vi "Begin.vi"(8 "error in":errorcluster) -> (0 "error out":errorcluster)   [LabVIEW 2015]
doc: "Called before other user functions, this VI is expected to open initial I/O refnums, load in file data, and do all program initialization. Notice that the <B>error out</B> terminal is simply used for data flow. Wiring it to other structures or subVIs ensures that this VI runs first."
uses:
  <vilib>/Rock Robotics/WPI/DriverStation/WPI_DriverStationRobotMode2.ctl
  <vilib>/Rock Robotics/WPI/Joystick/WPI_JoystickDeviceEnum.ctl
  <vilib>/Rock Robotics/SystemInterfaces/DIO/FPGA_DIOPWMChannel.ctl
  <vilib>/Rock Robotics/SystemInterfaces/DIO/FPGA_DIOChannel.ctl
  <vilib>/Rock Robotics/SystemInterfaces/DIO/FPGA_DIORelayChannel.ctl
  <vilib>/Rock Robotics/WPI/Camera/WPI_CameraExposure Values.ctl
  <vilib>/Rock Robotics/WPI/Camera/WPI_CameraWhite Balance Values.ctl
  <vilib>/Rock Robotics/WPI/Camera/WPI_CameraFrameRate.ctl
  <vilib>/Rock Robotics/WPI/Camera/WPI_CameraImageSize.ctl
  Robot Global Data.vi
  <vilib>/Rock Robotics/Network Tables/NT Write String Array.vi
  <vilib>/Rock Robotics/WPI/MotorControl/WPI_MotorControlOpen Talon.vi
  <vilib>/Rock Robotics/WPI/MotorControl/WPI_MotorControlOpen Victor.vi
  <vilib>/Rock Robotics/Network Tables/NT Write String.vi
  SubSystems/References/Refnums.vi
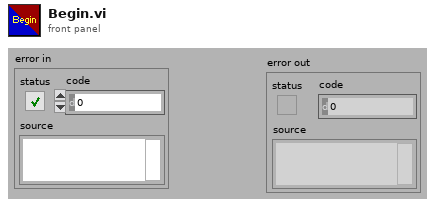
[diagram p1: front panel]
types:
  T1 = typedef "WPI_CameraImageSize.ctl" = enum16{"640x480", "320x240", "160x120", "Custom"}
  T2 = typedef "WPI_CameraFrameRate.ctl" = u32
  T3 = typedef "WPI_CameraExposure Values.ctl" = enum16{"Auto", "Flicker-free 50 Hz", "Flicker-free 60 Hz", "Hold current", "Custom"}
  T4 = typedef "WPI_CameraWhite Balance Values.ctl" = enum16{"Auto", "Fixed indoor", "Fixed outdoor 1", "Fixed outdoor 2", "Fixed fluorescent 1", "Fixed fluorescent 2", "Hold current", "Custom"}
  T5 = typedef "FPGA_DIORelayChannel.ctl" = enum8{"Relay 0", "Relay 1", "Relay 2", "Relay 3", "Invalid"}
  T6 = typedef "FPGA_DIOChannel.ctl" = enum8{"DIO 0", "DIO 1", "DIO 2", "DIO 3", "DIO 4", "DIO 5", "DIO 6", "DIO 7", "DIO 8", "DIO 9", "DIO MXP 0", "DIO MXP 1", "DIO MXP 2", "DIO MXP 3", "DIO MXP 4", "DIO MXP 5", "DIO MXP 6", "DIO MXP 7", "DIO MXP 8", "DIO MXP 9", "DIO MXP 10", "DIO MXP 11", "DIO MXP 12", "DIO MXP 13", "DIO MXP 14", "DIO MXP 15", "Invalid"}
  T7 = typedef "WPI_JoystickDeviceEnum.ctl" = enum16{"USB 0", "USB 1", "USB 2", "USB 3", "USB 4", "USB 5"}
  T8 = typedef "FPGA_DIOPWMChannel.ctl" = enum8{"PWM 0", "PWM 1", "PWM 2", "PWM 3", "PWM 4", "PWM 5", "PWM 6", "PWM 7", "PWM 8", "PWM 9", "PWM MXP 0", "PWM MXP 1", "PWM MXP 2", "PWM MXP 3", "PWM MXP 4", "PWM MXP 5", "PWM MXP 6", "PWM MXP 7", "PWM MXP 8", "PWM MXP 9", "Invalid"}
  T9 = typedef "WPI_DriverStationRobotMode2.ctl" = enum16{"Autonomous Disabled", "Autonomous Enabled", "Teleop Disabled", "Teleop Enabled", "Disconnected", "Finish", "Test Disabled", "Test Enabled", "Emergency Stopped"}
  T10 = typedef "WPI_JoystickDevRef.ctl" = cluster{"Device":T7}
  T11 = typedef "WPI_MotorControlDeviceRef.ctl" = cluster{"DeviceStatus":errorcluster, "Type":T12, "PWM":cluster{"PWM Channel":T8, "DeadBand":T13}, "CAN":cluster{"Device Number":u8, "Control Mode":T14, "Semaphore":T15, "Max Vout":dbl, "TalonSRX Control Mode":T16}, "Invert":bool}
  T12 = typedef "WPI_MotorControlType.ctl" = enum16{"PWM", "CAN", "CANTalonSRX"}
  T13 = typedef "WPI_PWMDeadband.ctl" = cluster{"Name":string, "maxPositivePwm":i32, "minPositivePwm":i32, "centerPwm":i32, "maxNegativePwm":i32, "minNegativePwm":i32, "angularRange":u16}
  T14 = typedef "WPI_CANJaguar_ControlMode.ctl" = enum8{"Percent VBus", "Current", "Speed", "Position", "Voltage"}
  T15 = typedef "Semaphore RefNum" = refnum<k1>
  T16 = typedef "WPI_CANTalonSRX_APIControlMode.ctl" = enum8{"Percent VBus", "Speed", "Position", "Slave", "Unchanged / Invalid", "Voltage Compensation", "Current", "Motion Profile"}
  T17 = typedef "WPI_RelayDevRef.ctl" = cluster{"DevStatus":errorcluster, "Relay Channel":T5, "Relay Direction":T18}
  T18 = typedef "WPI_RelayDirection.ctl" = enum16{"Both directions", "Forward only", "Reverse only"}
  T19 = typedef "WPI_CameraDevRef.ctl" = cluster{"Camera Address":string, "CameraStatus":errorcluster}
  T20 = typedef "WPI_DigitalInputDevRef.ctl" = cluster{"DevStatus":errorcluster, "DIO Channel":T6}
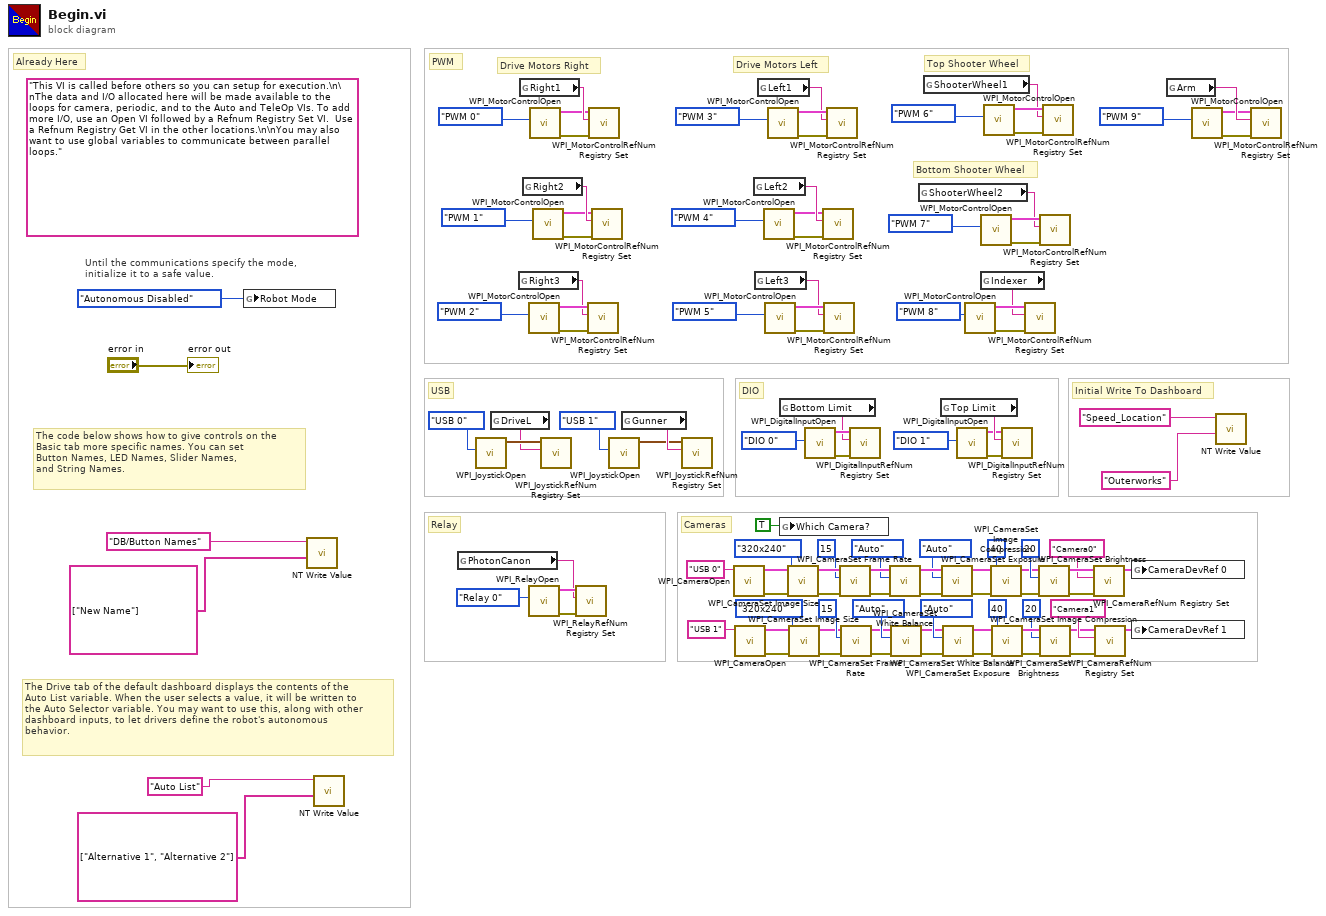
[diagram p0: block diagram]
diagram:
  (unwired) "This VI is called before others so you can setup for execution.\n\nThe data and I/O allocated here will be made available to the loops for camera, periodic, and to the Auto and TeleOp VIs. To add more I/O, use an Open VI followed by a Refnum Registry Set VI.  Use a Refnum Registry Get VI in the other locations.\n\nYou may also want to use global variables to communicate between parallel loops."
  # "Cameras"
  # "Initial Write To Dashboard"
  # "Bottom Shooter Wheel"
  # "Top Shooter Wheel"
  # "Drive Motors Left"
  # "Drive Motors Right"
  # "Relay"
  # "DIO"
  # "PWM"
  # "Already Here"
  # "USB"
  # "The Drive tab of the default dashboard displays the contents of the\nAuto List variable. When the user selects a value, it will be written to\nthe Auto Selector variable. You may want to use this, along with other\ndashboard inputs, to let drivers define the robot's autonomous\nbehavior."
  # "The code below shows how to give controls on the\nBasic tab more specific names. You can set\nButton Names, LED Names, Slider Names,\nand String Names."
  # "Until the communications specify the mode,\ninitialize it to a safe value."
  n1 = global write "Robot Global Data.vi" "Robot Mode"(WPI_DriverStationRobotMode2."Autonomous Disabled" ("Robot Mode")) -> ()
  n2 = call-poly <vilib>:"NT Write Value.vi"("String Array"=string[] ["New Name"], "Name"="DB/Button Names") -> ()  [unwired: 9 in, 1 out]
  n3 = call-poly <vilib>:"NT Write Value.vi"("String Array"=string[] ["Alternative 1", "Alternative 2"], "Name"="Auto List") -> ()  [unwired: 9 in, 1 out]
  n4 = global read "Refnums.vi" "PhotonCanon"() -> (w50:string)
  n5 = call <vilib>:"WPI_JoystickOpen.vi"("JoystickDevice"=WPI_JoystickDeviceEnum."USB 0") -> ("JoystickDevRef"=w107:T10)  [unwired: 10 in]
  n6 = global read "Refnums.vi" "DriveL"() -> (w106:string)
  n7 = global read "Refnums.vi" "Right3"() -> (w76:string)
  n8 = global read "Refnums.vi" "Right1"() -> (w84:string)
  n9 = global read "Refnums.vi" "Right2"() -> (w80:string)
  n10 = call-poly <vilib>:"WPI_MotorControlOpen.vi"("PWM Channel"=FPGA_DIOPWMChannel."PWM 2") -> ("error out"=w75:errorcluster, "MotorControlDeviceRef"=w77:T11)  [unwired: 9 in]
  n11 = call <vilib>:"WPI_RelayOpen.vi"("Relay Channel"=FPGA_DIORelayChannel."Relay 0") -> ("error out"=w52:errorcluster, "RelayDevRef"=w51:T17)  [unwired: 9 in]
  n12 = call-poly <vilib>:"WPI_MotorControlOpen.vi"("PWM Channel"=FPGA_DIOPWMChannel."PWM 0") -> ("error out"=w81:errorcluster, "MotorControlDeviceRef"=w83:T11)  [unwired: 9 in]
  n13 = call-poly <vilib>:"WPI_MotorControlOpen.vi"("PWM Channel"=FPGA_DIOPWMChannel."PWM 1") -> ("error out"=w78:errorcluster, "MotorControlDeviceRef"=w79:T11)  [unwired: 9 in]
  n14 = call <vilib>:"WPI_JoystickRefNum Registry Set.vi"("refnum name"=w106, "JoystickDevRef"=w107) -> ()  [unwired: 8 in, 2 out]
  n15 = call <vilib>:"WPI_RelayRefNum Registry Set.vi"("error in (no error)"=w52, "refnum name"=w50, "RelayDevRef"=w51) -> ()  [unwired: 7 in, 2 out]
  n16 = call <vilib>:"WPI_MotorControlRefNum Registry Set.vi"("error in (no error)"=w75, "refnum name"=w76, "MotorControlDevRef"=w77) -> ()  [unwired: 7 in, 2 out]
  n17 = call <vilib>:"WPI_MotorControlRefNum Registry Set.vi"("error in (no error)"=w81, "refnum name"=w84, "MotorControlDevRef"=w83) -> ()  [unwired: 7 in, 2 out]
  n18 = call <vilib>:"WPI_MotorControlRefNum Registry Set.vi"("error in (no error)"=w78, "refnum name"=w80, "MotorControlDevRef"=w79) -> ()  [unwired: 7 in, 2 out]
  n19 = call <vilib>:"WPI_JoystickOpen.vi"("JoystickDevice"=WPI_JoystickDeviceEnum."USB 1") -> ("JoystickDevRef"=w62:T10)  [unwired: 10 in]
  n20 = global read "Refnums.vi" "Gunner"() -> (w63:string)
  n21 = call <vilib>:"WPI_JoystickRefNum Registry Set.vi"("refnum name"=w63, "JoystickDevRef"=w62) -> ()  [unwired: 8 in, 2 out]
  n22 = call <vilib>:"WPI_CameraOpen.vi"("Camera Address"="USB 0") -> ("error out"=w37:errorcluster, "CameraDevRef"=w38:T19)  [unwired: 1 in, 8 out]
  n23 = call <vilib>:"WPI_CameraOpen.vi"("Camera Address"="USB 1") -> ("error out"=w14:errorcluster, "CameraDevRef"=w13:T19)  [unwired: 1 in, 8 out]
  n24 = global read "Refnums.vi" "Left2"() -> (w89:string)
  n25 = global read "Refnums.vi" "Left3"() -> (w85:string)
  n26 = global read "Refnums.vi" "Left1"() -> (w90:string)
  n27 = call-poly <vilib>:"WPI_MotorControlOpen.vi"("PWM Channel"=FPGA_DIOPWMChannel."PWM 4") -> ("error out"=w87:errorcluster, "MotorControlDeviceRef"=w88:T11)  [unwired: 9 in]
  n28 = call-poly <vilib>:"WPI_MotorControlOpen.vi"("PWM Channel"=FPGA_DIOPWMChannel."PWM 5") -> ("error out"=w82:errorcluster, "MotorControlDeviceRef"=w86:T11)  [unwired: 9 in]
  n29 = call-poly <vilib>:"WPI_MotorControlOpen.vi"("PWM Channel"=FPGA_DIOPWMChannel."PWM 3") -> ("error out"=w91:errorcluster, "MotorControlDeviceRef"=w92:T11)  [unwired: 9 in]
  n30 = global read "Refnums.vi" "Bottom Limit"() -> (w59:string)
  n31 = global write "Robot Global Data.vi" "Which Camera?"(TRUE ("Which Camera?")) -> ()
  n32 = call <vilib>:"WPI_CameraSet Image Size.vi"("error in (no error)"=w37, "Image Size"=WPI_CameraImageSize."320x240", "CameraDevRef"=w38) -> ("error out"=w36:errorcluster, "CameraDevRef Out"=w39:T19)  [unwired: 1 in, 6 out]
  n33 = call <vilib>:"WPI_CameraSet Image Size.vi"("error in (no error)"=w14, "Image Size"=WPI_CameraImageSize."320x240", "CameraDevRef"=w13) -> ("error out"=w15:errorcluster, "CameraDevRef Out"=w12:T19)  [unwired: 1 in, 6 out]
  n34 = call <vilib>:"WPI_DigitalInputOpen.vi"("DIO Channel"=FPGA_DIOChannel."DIO 0") -> ("error out"=w61:errorcluster, "DigitalInputDevRef"=w60:T20)  [unwired: 9 in]
  n35 = call <vilib>:"WPI_MotorControlRefNum Registry Set.vi"("error in (no error)"=w87, "refnum name"=w89, "MotorControlDevRef"=w88) -> ()  [unwired: 7 in, 2 out]
  n36 = call <vilib>:"WPI_MotorControlRefNum Registry Set.vi"("error in (no error)"=w82, "refnum name"=w85, "MotorControlDevRef"=w86) -> ()  [unwired: 7 in, 2 out]
  n37 = call <vilib>:"WPI_MotorControlRefNum Registry Set.vi"("error in (no error)"=w91, "refnum name"=w90, "MotorControlDevRef"=w92) -> ()  [unwired: 7 in, 2 out]
  n38 = call <vilib>:"WPI_CameraSet Frame Rate.vi"("error in (no error)"=w36, "Frame Rate (fps)"=T2 15, "CameraDevRef"=w39) -> ("error out"=w35:errorcluster, "CameraDevRef Out"=w41:T19)  [unwired: 7 out]
  n39 = call <vilib>:"WPI_CameraSet Frame Rate.vi"("error in (no error)"=w15, "Frame Rate (fps)"=T2 15, "CameraDevRef"=w12) -> ("error out"=w16:errorcluster, "CameraDevRef Out"=w10:T19)  [unwired: 7 out]
  n40 = call <vilib>:"WPI_DigitalInputRefNum Registry Set.vi"("error in (no error)"=w61, "refnum name"=w59, "DigitalInputDevRef"=w60) -> ()  [unwired: 7 in, 2 out]
  n41 = call <vilib>:"WPI_CameraSet White Balance.vi"("error in (no error)"=w35, "White Balance"=WPI_CameraWhite_Balance_Values."Auto", "CameraDevRef"=w41) -> ("error out"=w34:errorcluster, "CameraDevRef Out"=w40:T19)  [unwired: 1 in, 6 out]
  n42 = call <vilib>:"WPI_CameraSet White Balance.vi"("error in (no error)"=w16, "White Balance"=WPI_CameraWhite_Balance_Values."Auto", "CameraDevRef"=w10) -> ("error out"=w17:errorcluster, "CameraDevRef Out"=w11:T19)  [unwired: 1 in, 6 out]
  n43 = global read "Refnums.vi" "ShooterWheel2"() -> (w100:string)
  n44 = global read "Refnums.vi" "ShooterWheel1"() -> (w97:string)
  n45 = global read "Refnums.vi" "Top Limit"() -> (w56:string)
  n46 = call <vilib>:"WPI_CameraSet Exposure.vi"("error in (no error)"=w34, "Exposure"=WPI_CameraExposure_Values."Auto", "CameraDevRef"=w40) -> ("error out"=w33:errorcluster, "CameraDevRef Out"=w43:T19)  [unwired: 1 in, 6 out]
  n47 = call <vilib>:"WPI_CameraSet Exposure.vi"("error in (no error)"=w17, "Exposure"=WPI_CameraExposure_Values."Auto", "CameraDevRef"=w11) -> ("error out"=w18:errorcluster, "CameraDevRef Out"=w8:T19)  [unwired: 1 in, 6 out]
  n48 = call <vilib>:"WPI_DigitalInputOpen.vi"("DIO Channel"=FPGA_DIOChannel."DIO 1") -> ("error out"=w54:errorcluster, "DigitalInputDevRef"=w55:T20)  [unwired: 9 in]
  n49 = call-poly <vilib>:"WPI_MotorControlOpen.vi"("PWM Channel"=FPGA_DIOPWMChannel."PWM 8") -> ("error out"=w95:errorcluster, "MotorControlDeviceRef"=w94:T11)  [unwired: 9 in]
  n50 = call-poly <vilib>:"WPI_MotorControlOpen.vi"("PWM Channel"=FPGA_DIOPWMChannel."PWM 7") -> ("error out"=w102:errorcluster, "MotorControlDeviceRef"=w101:T11)  [unwired: 9 in]
  n51 = global read "Refnums.vi" "Indexer"() -> (w93:string)
  n52 = call-poly <vilib>:"WPI_MotorControlOpen.vi"("PWM Channel"=FPGA_DIOPWMChannel."PWM 6") -> ("error out"=w99:errorcluster, "MotorControlDeviceRef"=w98:T11)  [unwired: 9 in]
  n53 = call <vilib>:"WPI_CameraSet Image Compression.vi"("error in (no error)"=w33, "Compression"=40, "CameraDevRef"=w43) -> ("error out"=w32:errorcluster, "CameraDevRef Out"=w42:T19)  [unwired: 7 out]
  n54 = call <vilib>:"WPI_CameraSet Image Compression.vi"("error in (no error)"=w18, "Compression"=40, "CameraDevRef"=w8) -> ("error out"=w19:errorcluster, "CameraDevRef Out"=w9:T19)  [unwired: 7 out]
  n55 = call <vilib>:"WPI_DigitalInputRefNum Registry Set.vi"("error in (no error)"=w54, "refnum name"=w56, "DigitalInputDevRef"=w55) -> ()  [unwired: 7 in, 2 out]
  n56 = call <vilib>:"WPI_MotorControlRefNum Registry Set.vi"("error in (no error)"=w95, "refnum name"=w93, "MotorControlDevRef"=w94) -> ()  [unwired: 7 in, 2 out]
  n57 = call <vilib>:"WPI_CameraSet Brightness.vi"("error in (no error)"=w32, "Brightness"=20, "CameraDevRef"=w42) -> ("error out"=w31:errorcluster, "CameraDevRef Out"=w47:T19)  [unwired: 7 out]
  n58 = call <vilib>:"WPI_MotorControlRefNum Registry Set.vi"("error in (no error)"=w102, "refnum name"=w100, "MotorControlDevRef"=w101) -> ()  [unwired: 7 in, 2 out]
  n59 = call <vilib>:"WPI_CameraSet Brightness.vi"("error in (no error)"=w19, "Brightness"=20, "CameraDevRef"=w9) -> ("error out"=w20:errorcluster, "CameraDevRef Out"=w4:T19)  [unwired: 7 out]
  n60 = call <vilib>:"WPI_MotorControlRefNum Registry Set.vi"("error in (no error)"=w99, "refnum name"=w97, "MotorControlDevRef"=w98) -> ()  [unwired: 7 in, 2 out]
  n61 = call <vilib>:"WPI_CameraRefNum Registry Set.vi"("error in (no error)"=w31, "refnum name"="Camera0", "CameraDevRef"=w47) -> ("CameraDevRef"=w3:T19)  [unwired: 1 in, 7 out]
  n62 = call <vilib>:"WPI_CameraRefNum Registry Set.vi"("error in (no error)"=w20, "refnum name"="Camera1", "CameraDevRef"=w4) -> ("CameraDevRef"=w2:T19)  [unwired: 1 in, 7 out]
  n63 = global write "Robot Global Data.vi" "CameraDevRef 0"(w3) -> ()
  n64 = global write "Robot Global Data.vi" "CameraDevRef 1"(w2) -> ()
  n65 = global read "Refnums.vi" "Arm"() -> (w66:string)
  n66 = call-poly <vilib>:"WPI_MotorControlOpen.vi"("PWM Channel"=FPGA_DIOPWMChannel."PWM 9") -> ("error out"=w67:errorcluster, "MotorControlDeviceRef"=w65:T11)  [unwired: 9 in]
  n67 = call-poly <vilib>:"NT Write Value.vi"("String"="Outerworks", "Name"="Speed_Location") -> ()  [unwired: 9 in, 1 out]
  n68 = call <vilib>:"WPI_MotorControlRefNum Registry Set.vi"("error in (no error)"=w67, "refnum name"=w66, "MotorControlDevRef"=w65) -> ()  [unwired: 7 in, 2 out]
  "error out" <- "error in"
